vi "ErrCheck_Balanced Paranthesis.vi"(8 "Error In":errorcluster, 11 "Macro Command String IN":string="LOOP.Start\t(loop.iterations,3.000);") -> (0 "Error Out":errorcluster, 3 "Unbalanced Paranthesis or Commas?":bool)   [LabVIEW 2012]
doc: "SciScan 1.2 160622"
uses:
  <vilib>/Utility/error.llb/whitespace.ctl
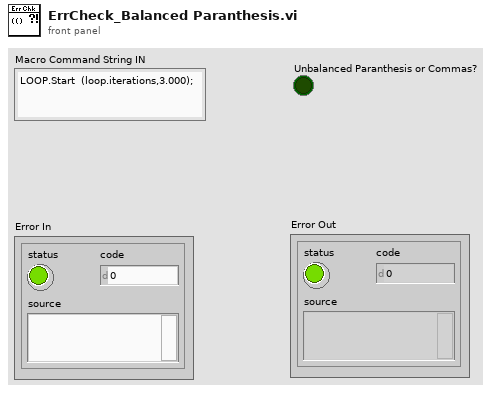
[diagram p1: front panel]
types:
  T1 = typedef "whitespace.ctl" = u16
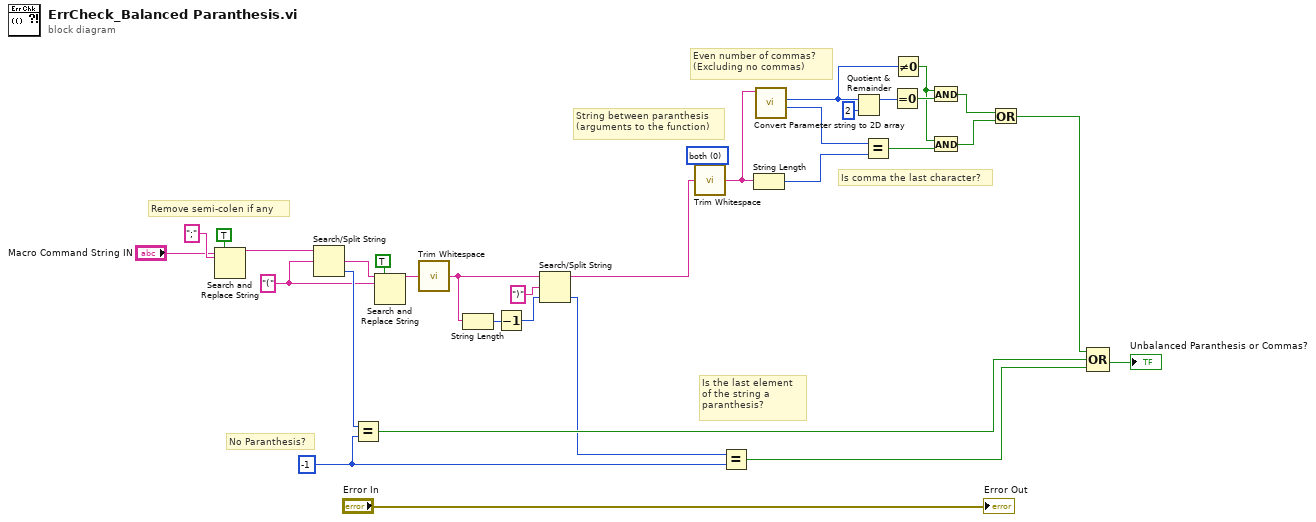
[diagram p0: block diagram]
diagram:
  w22 = T1 0 items=["both", "start of string", "end of string"] ("location (both)")
  w31 = -1 ("y")
  w25 = "(" ("search string/char (-)")
  # "Remove semi-colen if any"
  # "Is the last element of the string a paranthesis?"
  # "String between paranthesis\n(arguments to the function)"
  # "Is comma the last character?"
  # "Even number of commas?\n(Excluding no commas)"
  # "No Paranthesis?"
  n1 = Search and Replace String(replace all?=TRUE ("replace all? (F)"), input string="Macro Command String IN", search string=";") -> (result string=w4:string)  [unwired: 5 in, 3 out]
  n2 = Search/Split String(string=w4, search string/char (-)=w25) -> (match + rest of string=w30:string, offset of match=w32:i32)  [unwired: 1 in, 1 out]
  n3 = Equal?(x=w32, y=w31) -> (x = y?=w27:bool)
  n4 = Search and Replace String(replace all?=TRUE ("replace all? (F)"), input string=w30, search string=w25) -> (result string=w23:string)  [unwired: 5 in, 3 out]
  n5 = call <vilib>:"Trim Whitespace.vi"("string"=w23) -> ("trimmed string"=w9:string)  [unwired: 1 in]
  n6 = String Length(string=w9) -> (length=w8:i32)
  n7 = Decrement(x=w8) -> (x-1=w7:i32)
  n8 = Search/Split String(string=w9, search string/char (-)=")", offset (0)=w7) -> (substring before match=w2:string, offset of match=w1:i32)  [unwired: 1 out]
  n9 = call <vilib>:"Trim Whitespace.vi"("string"=w2, "location (both)"=w22) -> ("trimmed string"=w19:string)
  n10 = Equal?(x=w1, y=w31) -> (x = y?=w26:bool)
  n11 = String Length(string=w19) -> (length=w16:i32)
  n12 = call "Convert Parameter string to 2D array.vi"("Parameter string IN (without paranthesis)"=w19) -> ("offset of last detected comma (0 if none)"=w18:i32, "Number of commas"=w15:i32)  [unwired: 7 in, 2 out]
  n13 = Quotient & Remainder(x=w15, y=2) -> (x-y*floor(x/y)=w20:i32)  [unwired: 1 out]
  n14 = Equal?(x=w18, y=w16) -> (x = y?=w12:bool)
  n15 = Equal To 0?(x=w20) -> (x = 0?=w14:bool)
  n16 = Not Equal To 0?(x=w15) -> (x != 0?=w11:bool)
  n17 = And(x=w11, y=w14) -> (x .and. y?=w13:bool)
  n18 = And(x=w11, y=w12) -> (x .and. y?=w10:bool)
  n19 = Or(x=w13, y=w10) -> (x .or. y?=w17:bool)
  n20 = Compound Arithmetic op=OR(w17, w27, w26) -> (→"Unbalanced Paranthesis or Commas?":bool)
  "Error Out" <- "Error In"
